vi "Calibrations_Load.vi"(8 "error in":errorcluster, 11 "Subsystem":string="MySubsystem") -> (0 "error out":errorcluster)   [LabVIEW 2020]
uses:
  <vilib>/Utility/config.llb/NI_LVConfig.lvlib
  <vilib>/Utility/Data Type/NI_Data Type.lvlib
  <vilib>/Rock Robotics/Network Tables/NT Write Boolean.vi
  <vilib>/Utility/config.llb/Read Key (Boolean).vi
  <vilib>/Utility/config.llb/Read Key (String).vi
  <vilib>/Rock Robotics/Network Tables/NT Write String.vi
  <vilib>/Utility/config.llb/Read Key (I32).vi
  <vilib>/Rock Robotics/Network Tables/NT Write Number.vi
  <vilib>/Utility/config.llb/Read Key (Double).vi
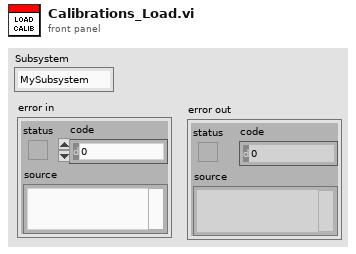
[diagram p1: front panel]
types:
  T1 = typedef "NI_LVConfig.lvlib/Config Data RefNum.ctl" = refnum<k1>
  T2 = typedef "NI_Data Type.lvlib/Data Type.ctl" = enum8{"Invalid Type", "Void", "I8", "I16", "I32", "I64", "U8", "U16", "U32", "U64", "Single Float", "Double Float", "Extended Float", "Single Complex", "Double Complex", "Extended Complex", "Enum U8", "Enum U16", "Enum U32", "Enum U64", "Single Float With Unit", "Double Float With Unit", "Extended Float With Unit", "Single Complex with Unit", "Double Complex with Unit", "Extended Complex with Unit", "Boolean", "String", "Path", "Picture", "Tag", "Array", "Cluster", "Variant", "LV Variant", "Waveform", "Timestamp", "Digital Waveform", "Digital Data", "ExpressData", "Refnum", "External Data", "VI", "Poly VI", "LabVIEW Class Instance", "Fixed Point", "Set Collection", "Map Collection"}
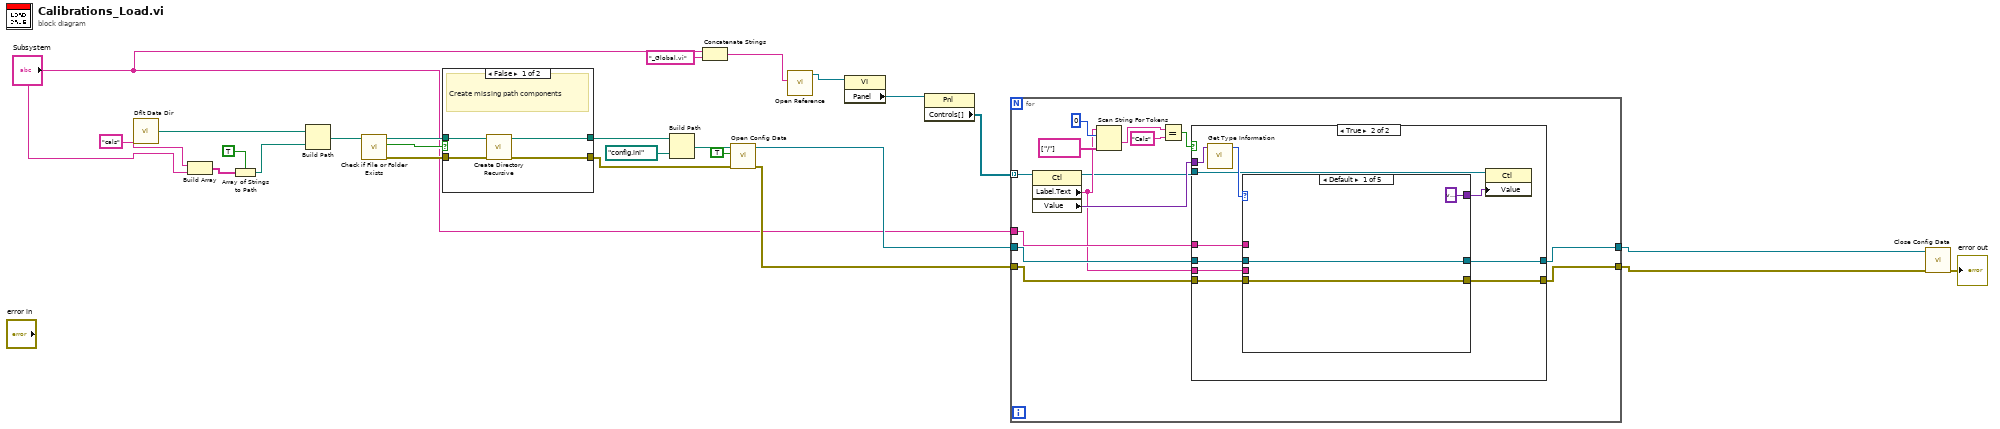
[diagram p0: block diagram]
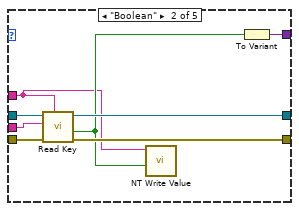
[diagram p3: hidden frame]
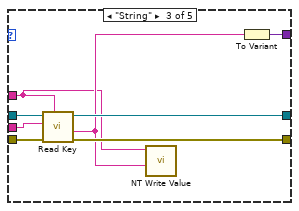
[diagram p4: hidden frame]
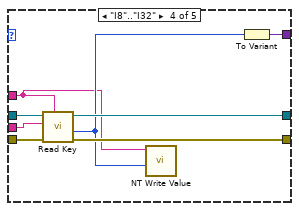
[diagram p5: hidden frame]
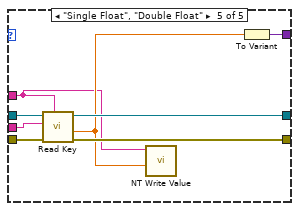
[diagram p6: hidden frame]
diagram:
  n1 = call <vilib>:"Dflt Data Dir.vi"() -> ("App:Default Data Directory"=w25:path)
  n2 = Build Array("cals" ("string"), "Subsystem") -> (w4:string[])
  n3 = Array of Strings to Path(0:w4, 1:TRUE ("relative")) -> (2:w3:path)
  n4 = Build Path(base path=w25, name or relative path=w3) -> (appended path=w24:path)
  n5 = call <vilib>:"Check if File or Folder Exists.vi"("path"=w24) -> ("error out"=w21:errorcluster, "file or folder exists?"=w23:bool, "dup path"=w22:path)  [unwired: 8 in]
  n6 = case shown="False" w23 {
    tunnel: w22 -> [w29 w31]
    tunnel: w21 -> [w28 w30]
    tunnel: [w27 w31] -> w20
    tunnel: [w26 w30] -> w16
    frame False {
      # "Create missing path components"
      n7 = call <vilib>:"Create Directory Recursive.vi"("error in (no error)"=w28, "directory"=w29) -> ("error out"=w26:errorcluster, "directory copy"=w27:path)  [unwired: 3 in, 1 out]
    }
    frame True {
      # "Bypass"
    }
  }
  n8 = Build Path(base path=w20, name or relative path=path "config.ini") -> (appended path=w18:path)
  n9 = Concatenate Strings("Subsystem", "_Global.vi" ("string")) -> (w14:string)
  n10 = call <vilib>:"Open Config Data.vi"("error in (no error)"=w16, "create file if necessary (T)"=TRUE, "configuration file path"=w18) -> ("error out"=w7:errorcluster, "refnum"=w10:T1)  [unwired: 6 in, 1 out]
  n11 = call "Open Reference.vi"("Front Panel VI Name"=w14) -> ("Front Panel Reference"=w13:refnum<vi>)  [unwired: 5 in, 1 out]
  n12 = property class="VI"(reference=w13) -> ("Panel"=w12:refnum<vi>)  [unwired: 1 in, 2 out]
  n13 = property class="Pnl"(reference=w12) -> ("Controls[]"=w11:refnum<vi>[])  [unwired: 1 in, 2 out]
  n14 = for {
    tunnel: w11 -> [w45] mode=indexing
    tunnel: w10 -> [w43]
    tunnel: "Subsystem" -> [w42]
    tunnel: [w41] -> w9
    tunnel: [w40] -> w8
    tunnel: w7 -> [w39]
    n15 = property class="Ctl"(reference=w45) -> (reference out=w32:refnum<vi>, "Label.Text"=w34:string, "Value"=w44:variant)  [unwired: 1 in, 1 out]
    n16 = Scan String For Tokens(6:string[] ["/"] ("operators (none)"), 8:0 ("offset"), 9:w34) -> (1:w33:string)  [unwired: 3 in, 3 out]
    n17 = Equal?(x=w33, y="Cals") -> (x = y?=w35:bool)
    n18 = case shown="True" w35 {
      tunnel: w44 -> [_ w56]
      tunnel: w43 -> [w47 w55]
      tunnel: w42 -> [_ w54]
      tunnel: [w47 w53] -> w41
      tunnel: [w46 w52] -> w40
      tunnel: w39 -> [w46 w51]
      tunnel: w34 -> [_ w50]
      tunnel: w32 -> [_ w49]
      frame False {
      }
      frame True {
        n19 = call <vilib>:"Get Type Information.vi"("variant"=w56) -> ("type"=w57:T2)  [unwired: 6 in, 4 out]
        n20 = case shown="Default" w57 {
          tunnel: w55 -> [w60 w68 w76 w84 w92]
          tunnel: w54 -> [_ w61 w69 w77 w85]
          tunnel: [w60 w67 w75 w83 w91] -> w53
          tunnel: [w59 w66 w74 w82 w90] -> w52
          tunnel: w51 -> [w59 w65 w73 w81 w89]
          tunnel: w50 -> [_ w64 w72 w80 w88]
          tunnel: [variant ("Variant") w63 w71 w79 w87] -> w48
          frame Default {
          }
          frame "Boolean" {
            n21 = call-poly <vilib>:"Read Key.vi"("section"=w61, "error in (no error)"=w65, "key"=w64, "refnum"=w68) -> ("error out"=w66:errorcluster, "value"=w62:bool, "refnum out"=w67:T1)  [unwired: 4 in, 1 out]
            n22 = call-poly <vilib>:"NT Write Value.vi"("Boolean"=w62, "Name"=w61) -> ()  [unwired: 9 in, 1 out]
            n23 = To Variant(anything=w62) -> (Variant=w63:variant)
          }
          frame "String" {
            n24 = call-poly <vilib>:"Read Key.vi"("section"=w69, "error in (no error)"=w73, "key"=w72, "refnum"=w76) -> ("error out"=w74:errorcluster, "value"=w70:string, "refnum out"=w75:T1)  [unwired: 4 in, 1 out]
            n25 = call-poly <vilib>:"NT Write Value.vi"("String"=w70, "Name"=w69) -> ()  [unwired: 9 in, 1 out]
            n26 = To Variant(anything=w70) -> (Variant=w71:variant)
          }
          frame "I8".."I32" {
            n27 = call-poly <vilib>:"Read Key.vi"("section"=w77, "error in (no error)"=w81, "key"=w80, "refnum"=w84) -> ("error out"=w82:errorcluster, "value"=w78:i32, "refnum out"=w83:T1)  [unwired: 4 in, 1 out]
            n28 = call-poly <vilib>:"NT Write Value.vi"("Numeric"=w78, "Name"=w77) -> ()  [unwired: 9 in, 1 out]
            n29 = To Variant(anything=w78) -> (Variant=w79:variant)
          }
          frame "Single Float", "Double Float" {
            n30 = call-poly <vilib>:"Read Key.vi"("section"=w85, "error in (no error)"=w89, "key"=w88, "refnum"=w92) -> ("error out"=w90:errorcluster, "value"=w86:dbl, "refnum out"=w91:T1)  [unwired: 4 in, 1 out]
            n31 = call-poly <vilib>:"NT Write Value.vi"("Numeric"=w86, "Name"=w85) -> ()  [unwired: 9 in, 1 out]
            n32 = To Variant(anything=w86) -> (Variant=w87:variant)
          }
        }
        n33 = property class="Ctl"(reference=w49, "Value"=w48) -> ()  [unwired: 1 in, 2 out]
      }
    }
  }
  n34 = call <vilib>:"Close Config Data.vi"("error in (no error)"=w8, "refnum"=w9) -> ("error out"=→"error out":errorcluster)  [unwired: 8 in, 1 out]
